vi "locateSettingsFile.vi"(8 "error in (no error)":errorcluster, 11 "VI Refnum in":refnum<vi>) -> (0 "error out":errorcluster, 2 "path":path, 3 "VI Refnum out":refnum<vi>)   [LabVIEW 2015, in "pdbm_tasks.lvlib"]
uses:
  pdbm_tasks.lvlib
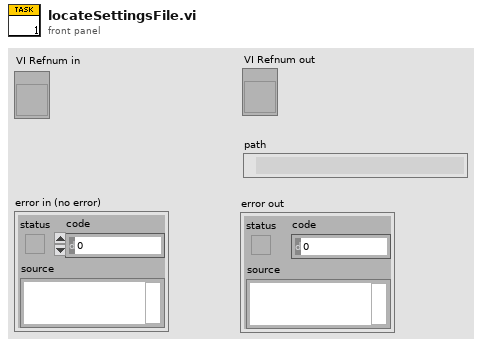
[diagram p1: front panel]
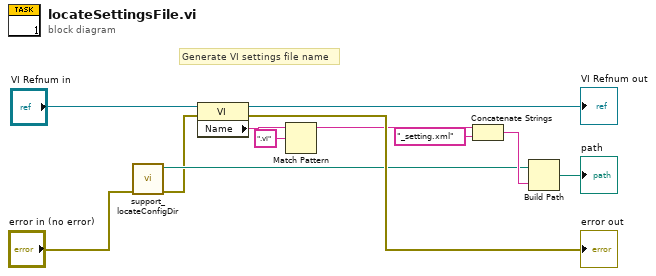
[diagram p0: block diagram]
diagram:
  # "Generate VI settings file name"
  n1 = call "support_locateConfigDir.vi"("error in (no error)"="error in (no error)") -> ("error IO"=w1:errorcluster, "Config path"=w3:path)  [unwired: 9 in]
  n2 = property class="VI"(reference="VI Refnum in", error in=w1) -> (reference out=→"VI Refnum out":refnum<vi>, error out=→"error out":errorcluster, "Name"=w6:string)
  n3 = Match Pattern(string=w6, regular expression=".vi") -> (before substring=w4:string)  [unwired: 1 in, 3 out]
  n4 = Concatenate Strings(w4, "_setting.xml" ("string")) -> (w10:string)
  n5 = Build Path(base path=w3, name or relative path=w10) -> (appended path=→"path":path)
